vi "Get Table.vi"(8 "error in (no error)":errorcluster, 11 "Panel Form Controller in":refnum<class "Panel Form Controller.lvclass">) -> (0 "error out":errorcluster, 2 "Table":refnum<class "Basic Table.lvclass">, 3 "Panel Form Controller out":refnum<class "Panel Form Controller.lvclass">)   [LabVIEW 2020, in "Panel Form Controller.lvlib" / "Panel Form Controller.lvclass"]
uses:
  Panel Form Controller.lvclass
  Database OOP/Table Libraries/Basic Table/Basic Table Class/Basic Table.lvclass
  Panel Form Controller.lvclass/Panel Form Controller.ctl
  Database OOP/Table Libraries/Basic Form/Basic Form.lvclass
  C:/Users/User/Desktop/Raman Program/Database OOP/source/Database OOP/Table Libraries/Basic Table/Basic Table Class/Basic Table.lvclass
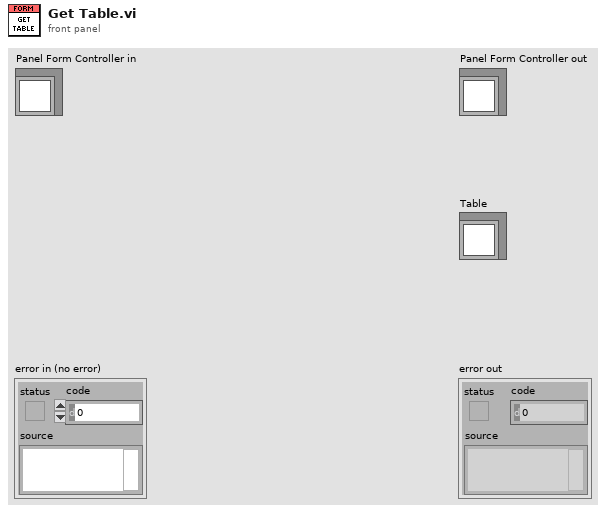
[diagram p1: front panel]
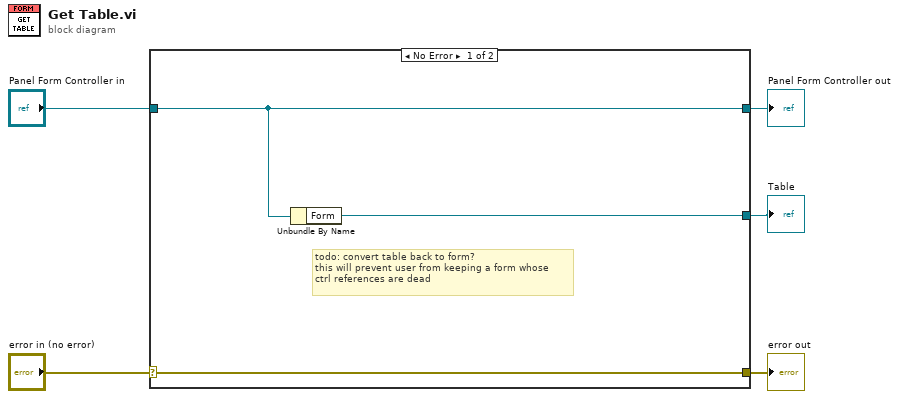
[diagram p0: block diagram]
diagram:
  n1 = case shown="No Error" "error in (no error)" {
    selector: "error in (no error)" -> [w8 w10]
    tunnel: [w8 w10] -> w4
    tunnel: [w7 w9] -> w2
    tunnel: "Panel Form Controller in" -> [w7 w9]
    tunnel: [w6 _] -> w1
    frame No Error {
      # "todo: convert table back to form?\nthis will prevent user from keeping a form whose\nctrl references are dead"
      n2 = Unbundle By Name(w7) -> ("Form"=w6:refnum<class "Basic Form.lvclass">)
    }
    frame Error {
    }
  }
  "error out" <- w4
  "Panel Form Controller out" <- w2
  "Table" <- w1
